vi "Target - File Management.vi"(5 "Authentication":T1={"User"="admin", "Password"="ptauto"}, 6 "Index":i32[](array[numeric]), 7 "Actions":T2, 8 "error in":errorcluster, 9 "Windows directory":path=path "C:/Temp/WebDAV/Files Transferred", 10 "relative uri":string="/home/lvuser/natinst/LabVIEW Data/Application Files", 11 "target address":string) -> (0 "error out":errorcluster, 1 "Folders":string[](array[string]), 2 "Files":string[][](array[string]))   [LabVIEW 2020]
uses:
  <vilib>/WebDAVClient/Advanced/FileInfo.ctl
  EPIT VI Factory/VI Factory EPIT  Source/SW/Reuse/WebDAV/File Actions.ctl
  EPIT VI Factory/VI Factory EPIT  Source/SW/Reuse/WebDAV/WebDAV Authentication.ctl
  <vilib>/WebDAVClient/Advanced/SessionHandle.ctl
  <vilib>/WebDAVClient/Advanced/Get File.vi
  <vilib>/WebDAVClient/NI_WebDAV.lvlib
panel:
  out "file list":T3[](array[typedef])
  out "directory list":T3[](array[typedef])
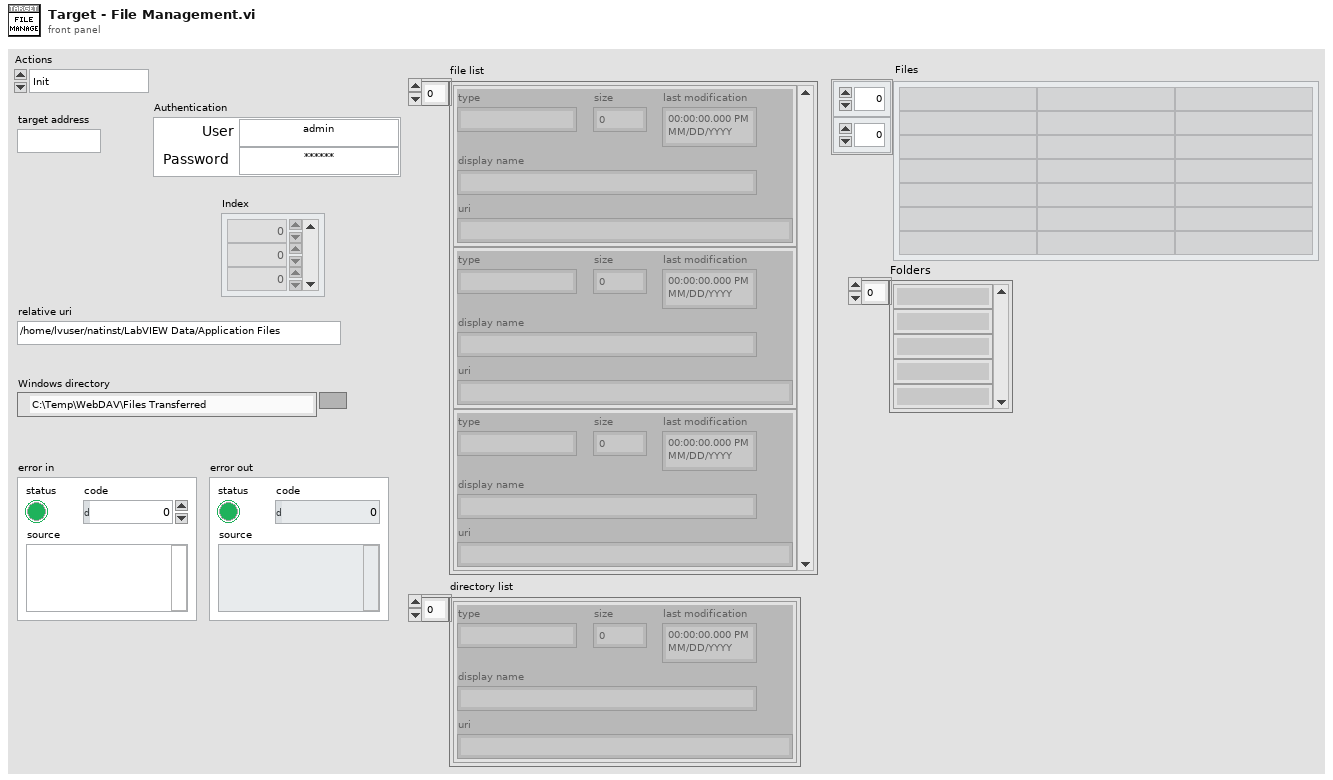
[diagram p1: front panel]
types:
  T1 = typedef "WebDAV Authentication.ctl" = cluster{"User":string, "Password":string}
  T2 = typedef "File Actions.ctl" = enum16{"Init", "Get All", "Get Selected", "Delete All", "Delete Selected", "Close"}
  T3 = typedef "NI_WebDAV.lvlib/FileInfo.ctl" = cluster{"type":string, "size":u64, "last modification":timestamp, "display name":string, "uri":string}
  T4 = typedef "NI_WebDAV.lvlib/SessionHandle.ctl" = refnum<k1>
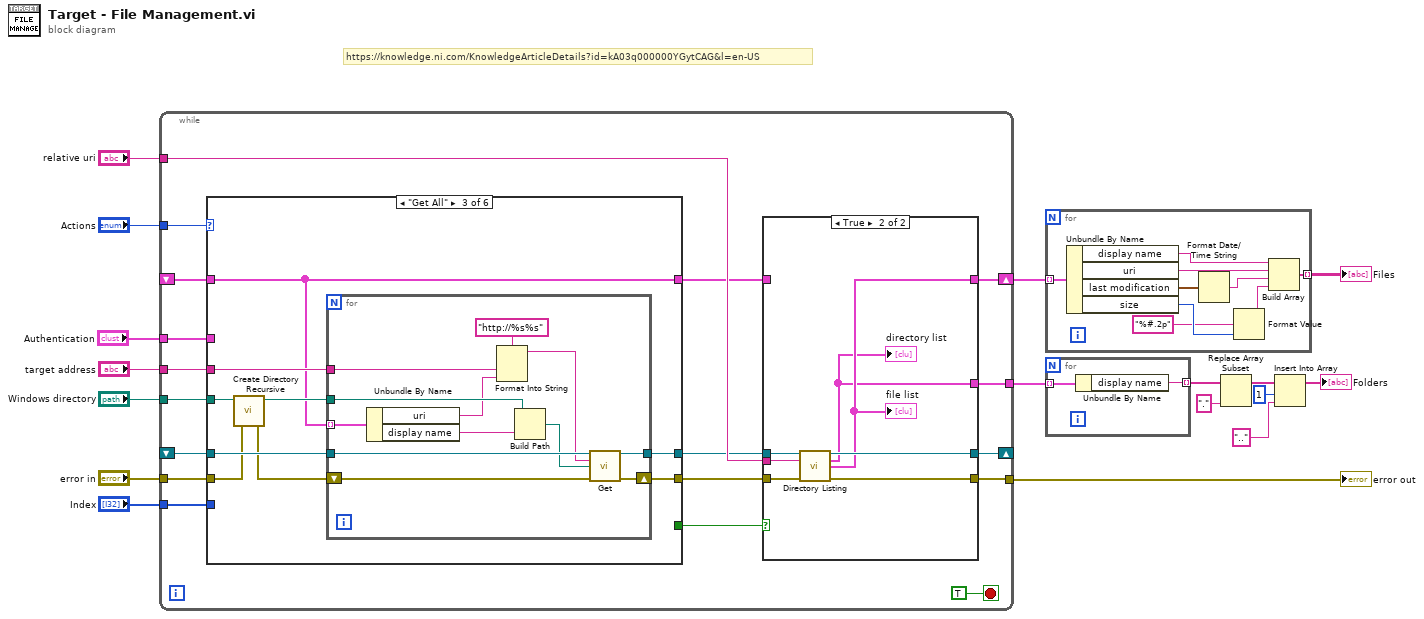
[diagram p0: block diagram]
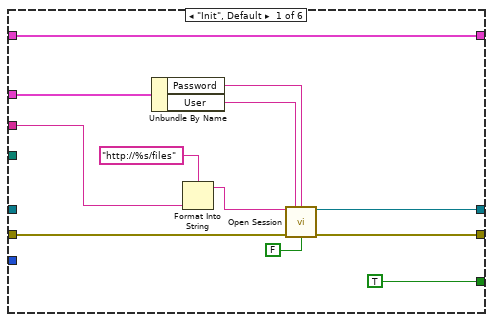
[diagram p2: hidden frame]
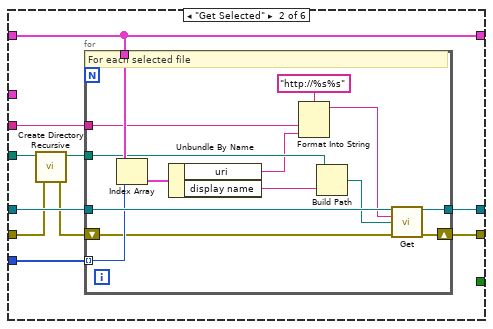
[diagram p3: hidden frame]
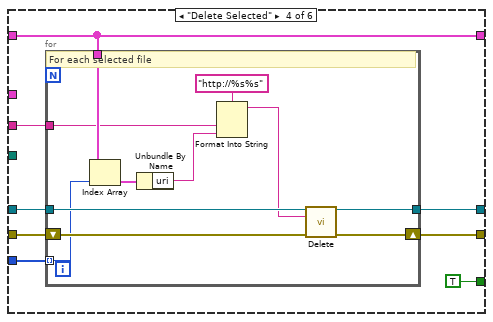
[diagram p4: hidden frame]
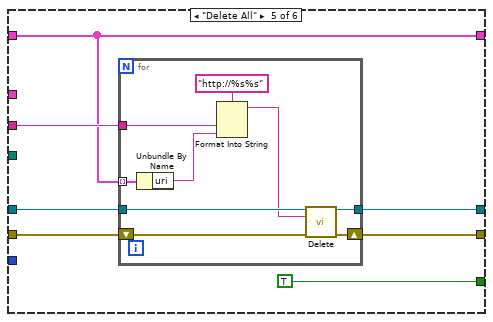
[diagram p5: hidden frame]
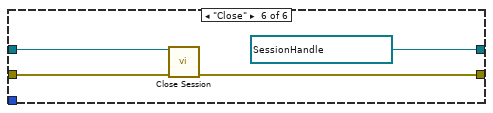
[diagram p6: hidden frame]
diagram:
  # "https://knowledge.ni.com/KnowledgeArticleDetails?id=kA03q000000YGytCAG&l=en-US"
  n1 = while {
    tunnel: "error in" -> [w33]
    tunnel: [w24] -> w16
    shift-right: [w22] -> w17
    shift-left: _ -> [w32]
    shift-right: [w25] -> _
    shift-left: _ -> [w31]
    tunnel: "Windows directory" -> [w30]
    tunnel: "Actions" -> [w34]
    tunnel: "Index" -> [w29]
    tunnel: "relative uri" -> [w27]
    tunnel: "target address" -> [w20]
    tunnel: [w19] -> w8
    tunnel: "Authentication" -> [w18]
    stop <- TRUE stop-if-true
    n2 = case shown="\"Get All\"" w34 {
      tunnel: w33 -> [w44 w51 w76 w100 w118 w131]
      tunnel: [w43 w56 w79 w98 w116 w130] -> w28
      tunnel: [w42 w55 w78 w97 w115 w128] -> w26
      tunnel: [w40 w53 w72 w95 w112 _] -> w21
      tunnel: w32 -> [w40 w53 w72 w95 w112 _]
      tunnel: w31 -> [_ w57 w80 w99 w117 w129]
      tunnel: w30 -> [_ w52 w77 _ _ _]
      tunnel: w29 -> [_ w54 _ w94 _ _]
      tunnel: [TRUE _ _ TRUE TRUE _] -> w23
      tunnel: w20 -> [w39 w48 w73 w93 w113 _]
      tunnel: w18 -> [w38 _ _ _ _ _]
      frame "Init", Default {
        n3 = Unbundle By Name(w38) -> ("Password"=w37:string, "User"=w36:string)
        n4 = Format Into String(format string="http://%s/files", w39) -> (resulting string=w47:string)  [unwired: 2 in, 1 out]
        n5 = call <vilib>:"Open Session.vi"("host uri prefix"=w47, "username"=w36, "password"=w37, "error in (no error)"=w44, "verify server?"=FALSE) -> ("session handle out"=w42:T4, "error out"=w43:errorcluster)  [unwired: 9 in]
      }
      frame "Get Selected" {
        n6 = call <vilib>:"Create Directory Recursive.vi"("error in (no error)"=w51, "directory"=w52) -> ("error out"=w50:errorcluster, "directory copy"=w49:path)  [unwired: 3 in, 1 out]
        n7 = for {
          tunnel: w57 -> [w71]
          tunnel: [w69] -> w55
          tunnel: w54 -> [w67] mode=indexing
          tunnel: w53 -> [w65]
          tunnel: w49 -> [w63]
          tunnel: w48 -> [w61]
          shift-right: [w70] -> w56
          shift-left: w50 -> [w64]
          # "For each selected file"
          n8 = Index Array(array=w65, index=w67) -> (element=w66:T3)
          n9 = Unbundle By Name(w66) -> ("uri"=w58:string, "display name"=w59:string)
          n10 = Format Into String(format string="http://%s%s", w61, w58) -> (resulting string=w60:string)  [unwired: 2 in, 1 out]
          n11 = Build Path(base path=w63, name or relative path=w59) -> (appended path=w68:path)
          n12 = call-poly <vilib>:"Get.vi"("session handle"=w71, "relative uri"=w60, "local file path"=w68, "error in (no error)"=w64) -> ("session handle out"=w69:T4, "error out"=w70:errorcluster)  [unwired: 9 in, 1 out]
        }
      }
      frame "Get All" {
        n13 = call <vilib>:"Create Directory Recursive.vi"("error in (no error)"=w76, "directory"=w77) -> ("error out"=w75:errorcluster, "directory copy"=w74:path)  [unwired: 3 in, 1 out]
        n14 = for {
          tunnel: w80 -> [w92]
          tunnel: [w90] -> w78
          tunnel: w74 -> [w87]
          tunnel: w73 -> [w85]
          shift-right: [w91] -> w79
          shift-left: w75 -> [w88]
          tunnel: w72 -> [w81] mode=indexing
          n15 = Unbundle By Name(w81) -> ("uri"=w82:string, "display name"=w83:string)
          n16 = Format Into String(format string="http://%s%s", w85, w82) -> (resulting string=w84:string)  [unwired: 2 in, 1 out]
          n17 = Build Path(base path=w87, name or relative path=w83) -> (appended path=w89:path)
          n18 = call-poly <vilib>:"Get.vi"("session handle"=w92, "relative uri"=w84, "local file path"=w89, "error in (no error)"=w88) -> ("session handle out"=w90:T4, "error out"=w91:errorcluster)  [unwired: 9 in, 1 out]
        }
      }
      frame "Delete Selected" {
        n19 = for {
          tunnel: w99 -> [w110]
          tunnel: [w108] -> w97
          tunnel: w95 -> [w107]
          tunnel: w94 -> [w105] mode=indexing
          tunnel: w93 -> [w102]
          shift-right: [w109] -> w98
          shift-left: w100 -> [w111]
          # "For each selected file"
          n20 = Index Array(array=w107, index=w105) -> (element=w106:T3)
          n21 = Unbundle By Name(w106) -> ("uri"=w103:string)
          n22 = Format Into String(format string="http://%s%s", w102, w103) -> (resulting string=w101:string)  [unwired: 2 in, 1 out]
          n23 = call <vilib>:"Delete.vi"("session handle"=w110, "relative uri"=w101, "error in (no error)"=w111) -> ("session handle out"=w108:T4, "error out"=w109:errorcluster)  [unwired: 11 in]
        }
      }
      frame "Delete All" {
        n24 = for {
          tunnel: w117 -> [w126]
          tunnel: [w124] -> w115
          tunnel: w113 -> [w121]
          shift-right: [w125] -> w116
          shift-left: w118 -> [w127]
          tunnel: w112 -> [w119] mode=indexing
          n25 = Unbundle By Name(w119) -> ("uri"=w122:string)
          n26 = Format Into String(format string="http://%s%s", w121, w122) -> (resulting string=w120:string)  [unwired: 2 in, 1 out]
          n27 = call <vilib>:"Delete.vi"("session handle"=w126, "relative uri"=w120, "error in (no error)"=w127) -> ("session handle out"=w124:T4, "error out"=w125:errorcluster)  [unwired: 11 in]
        }
      }
      frame "Close" {
        w128 = T4 refnum items=["Session NI_WebDAV"] ("session handle out")
        n28 = call <vilib>:"Close Session.vi"("session handle"=w129, "error in (no error)"=w131) -> ("error out"=w130:errorcluster)  [unwired: 13 in]
      }
    }
    n29 = case shown="True" w23 {
      tunnel: w28 -> [w132 w141]
      tunnel: w27 -> [_ w140]
      tunnel: w26 -> [w133 w139]
      tunnel: [w133 w138] -> w25
      tunnel: [w132 w137] -> w24
      tunnel: [w134 w136] -> w22
      tunnel: w21 -> [w134 _]
      tunnel: [_ w135] -> w19
      frame False {
      }
      frame True {
        n30 = call <vilib>:"Directory Listing.vi"("session handle"=w139, "relative uri"=w140, "error in (no error)"=w141) -> ("session handle out"=w138:T4, "directory list"=w135:T3[], "file list"=w136:T3[], "error out"=w137:errorcluster)  [unwired: 9 in]
        "directory list" <- w135
        "file list" <- w136
      }
    }
  }
  "error out" <- w16
  n31 = for {
    tunnel: w17 -> [w150] mode=indexing
    tunnel: [w147] -> w10 mode=indexing
    n32 = Unbundle By Name(w150) -> ("display name"=w149:string, "uri"=w148:string, "last modification"=w146:timestamp, "size"=w144:u64)
    n33 = Format Date/Time String(seconds (now)=w146) -> (date/time string=w145:string)  [unwired: 2 in]
    n34 = Format Value(format string="%#.2p", value (0)=w144) -> (output string=w142:string)  [unwired: 1 in]
    n35 = Build Array(w149, w148, w145, w142) -> (w147:string[])
  }
  "Files" <- w10
  n36 = for {
    tunnel: w8 -> [w152] mode=indexing
    tunnel: [w151] -> w7 mode=indexing
    n37 = Unbundle By Name(w152) -> ("display name"=w151:string)
  }
  n38 = Replace Array Subset(array=w7, new element="." ("new element/subarray")) -> (w6:string[])  [unwired: 1 in]
  n39 = Insert Into Array(array=w6, index=1, new element=".." ("new element/subarray")) -> (→"Folders":string[])
